vi "Collect_Info(V1.1).vi"(5 "HART ports":refnum<visa-resource-name>[](array[refnum]), 7 "485 Ports":refnum<visa-resource-name>[](array[refnum]), 10 "MODBUS Serial Parameters":T10={"Mode"=enum."RTU", "Default Slave Address"=111, "MODBUS timeout"=1000, "Baud Rate"=38400, "Parity"=0, "Flow Control"=0} {"Flow Control" items=["None", "XON/XOFF", "RTS/CTS", "XON/XOFF & RTS/CTS", "DTR/DSR", "XON/XOFF & DTR/DSR"]; "Parity" items=["None", "Odd", "Even", "Mark", "Space"]}) -> (1 "Read Completed":bool, 2 "Information":T11, 3 "Byte order":T7(ring))   [LabVIEW 2016]
uses:
  Controls/Control_Done.ctl
  Controls/Flow Tube Material.ctl
  Controls/mass flow unit codes.ctl
  Controls/Density Unit codes.ctl
  Controls/Temperature units.ctl
  Controls/Flow direction codes.ctl
  Controls/Information_tab_type.ctl
  Controls/Control_Sample.ctl
  OPC Server/MODBUS/MODBUS parameters type.ctl
  <vilib>/DeviceNet/VIAPI/subVIs/DnetIntfConfig.ctl
  OPC Server/Typedef/Array_of_Comm_mode_and_address_types.ctl
  OPC Server/Typedef/Comm_mode_and_address_type.ctl
  OPC Server/Typedef/Comm_mode_type_combo.ctl
  Controls/Control_EXIT.ctl
  Controls/ctrlCollectInfoStates.ctl
  Controls/ctrlCollectInfoData.ctl
  OPC Server/Protocol Class/Protocol.lvclass
  OPC Server/Typedef/comm_variable_definition.ctl
  OPC Server/MASTER_OPC.ctl
  OPC Server/Typedef/event var.ctl
  OPC Server/Typedef/Comm ui action type.ctl
  OPC Server/Typedef/Comm_State_enum.ctl
  OPC Server/Typedef/state var.ctl
  <vilib>/Utility/miscctls.llb/LVPointTypeDef.ctl
  OPC Server/MODBUS/MODBUS Class/MODBUS.lvclass
  C:/Application/Blackbox_US-Rabi--master/OPC Server/Protocol Class/Protocol.lvclass
  OPC Server/HART/HART Class/HART.lvclass
  OPC Server/Profibus/Profibus Class/Profibus.lvclass
  OPC Server/DeviceNET/DeviceNET Class/DeviceNET.lvclass
  OPC Server/Typedef/Protocol_enum_type.ctl
  <vilib>/DeviceNet/DeviceNetLIB.lvlib
panel:
  out "status":bool
  in  "Protocol selection\n(appended)":T1=[{"address"=111, "Mode"=0}, {"address"=0, "Mode"=2}] {"Mode" items=["MODBUS", "HART", ""]}
  in  "Done":T4
  in  "Read":T5
  in  "Batch Time":string
  in  "Pressure":string
  in  "Frequency":string
  in  "Test Gas":string
  in  "Stand Uncertainty":string
  in  "Customer PO":string
  in  "Fluid Temperature":string
  in  "Exit":T6
  in  "MDOT":string
  in  "Meter inlet static pressure (psia)":dbl
  in  "Fluid":string="H2O"
  in  "Product code*":string
  in  "Order number":string
  in  "Status *":enum32{"As found", "As left"}(radio)
  in  "Ref meter serial number*":string
  in  "Technician Name*":string
  in  "Customer Address":string
  in  "Customer Name":string
  in  "Interface Name":T8(ring)
  in  "DeviceNet Interface Configuration":T9={"interface MAC ID"=0, "baud rate"=enum."500000", "poll mode"=enum."Automatic"} {"interface MAC ID" max=63 step=1}
  in  "Profibus Baud rate":i32(listbox)=6
  in  "Profibus ResourceName":refnum<visa-resource-name>="PXI5::11::INSTR"
  in  "Test Comments":string
  out "Test date and time":string
  out "Meter Zero":string
  in  "Meter Nominal Flow Rate (kg/min)*":string
  in  "Meter Density Repeatability":string
  in  "Meter Density Accuracy":string
  in  "Meter Zero Stability (kg/min) *":string
  in  "Meter flow repeatability":string
  in  "Meter flow accuracy (%) *":string
  out "Frequency span":string
  out "Frequency flow rate":string
  out "Flow direction":T12 items=["Forward flow only", "Reverse flow only", "Bidirectiona flow", "Absolute forward/reverse", "Negate/Forward only", "Negate/Bidirectional"]
  out "Mass flow damping":string
  out "Mass flow cutoff":string
  out "Temperature Units":T13 items=["Degrees Celsius"=32, "Degrees Fahrenheit"=33, "Degrees Rankine"=34, "Degrees Kelvin"=35, ""=0]
  out "Density units":T14 items=["Specific gravity units"=90, "Grams/cubic centimeter"=91, "Kg/cubic meter"=92, "Pounds/US gallon"=93, "Pounds/cubic foot"=94, "Grams/milliliter"=95, "Kg/liter"=96, "Pounds/cubic inch"=98, "Short tons/cubic yard"=99, "Degrees Baume (heavy)"=102, "Degrees Baume (light)"=103, "Degrees API"=104]
  out "Mass flow units":T15 items=["Grams/second"=70, "Grams/minute"=71, "Grams/hour"=72, "Kg/second"=73, "Kg/minute"=74, "Kg/hour"=75, "Kg/day"=76, "Metric tons/minute"=77, "Metric tons/hour"=78, "Metric tons/day"=79, "Pounds/second"=80, "Pounds/minute"=81, "Pounds/hour"=82, "Pounds/day"=83, "Short tons/minute"=84, "Short tons/hour"=85, "Short tons/day"=86, "Long tons/hour"=87, "Long tons/day"=88, "Special"=253]
  out "Transmitter Model":string
  in  "Sensor Model #":string
  in  "Transmitter Serial Number":string
  out "Density Temp Coeff":string
  out "FD":string
  out "K2":string
  out "K1":string
  out "D2":string
  out "D1":string
  out "FCF":string
  in  "Temp Rating":string
  in  "Pressure Rating":string
  out "Sensor Serial Number":string
  out "Flow Tube Material":T16 items=["Hastelloy C-22"=3, "Monel"=4, "Tantalum"=5, "Titanium"=6, "316L Stainless Steel"=19, "Inconel"=23, "Unknown"=252, "Special"=253]
  in  "Size":string
  out "Header":string="CUSTOMER INFORMATION"
  # "Customer Information"
  # "*Required"
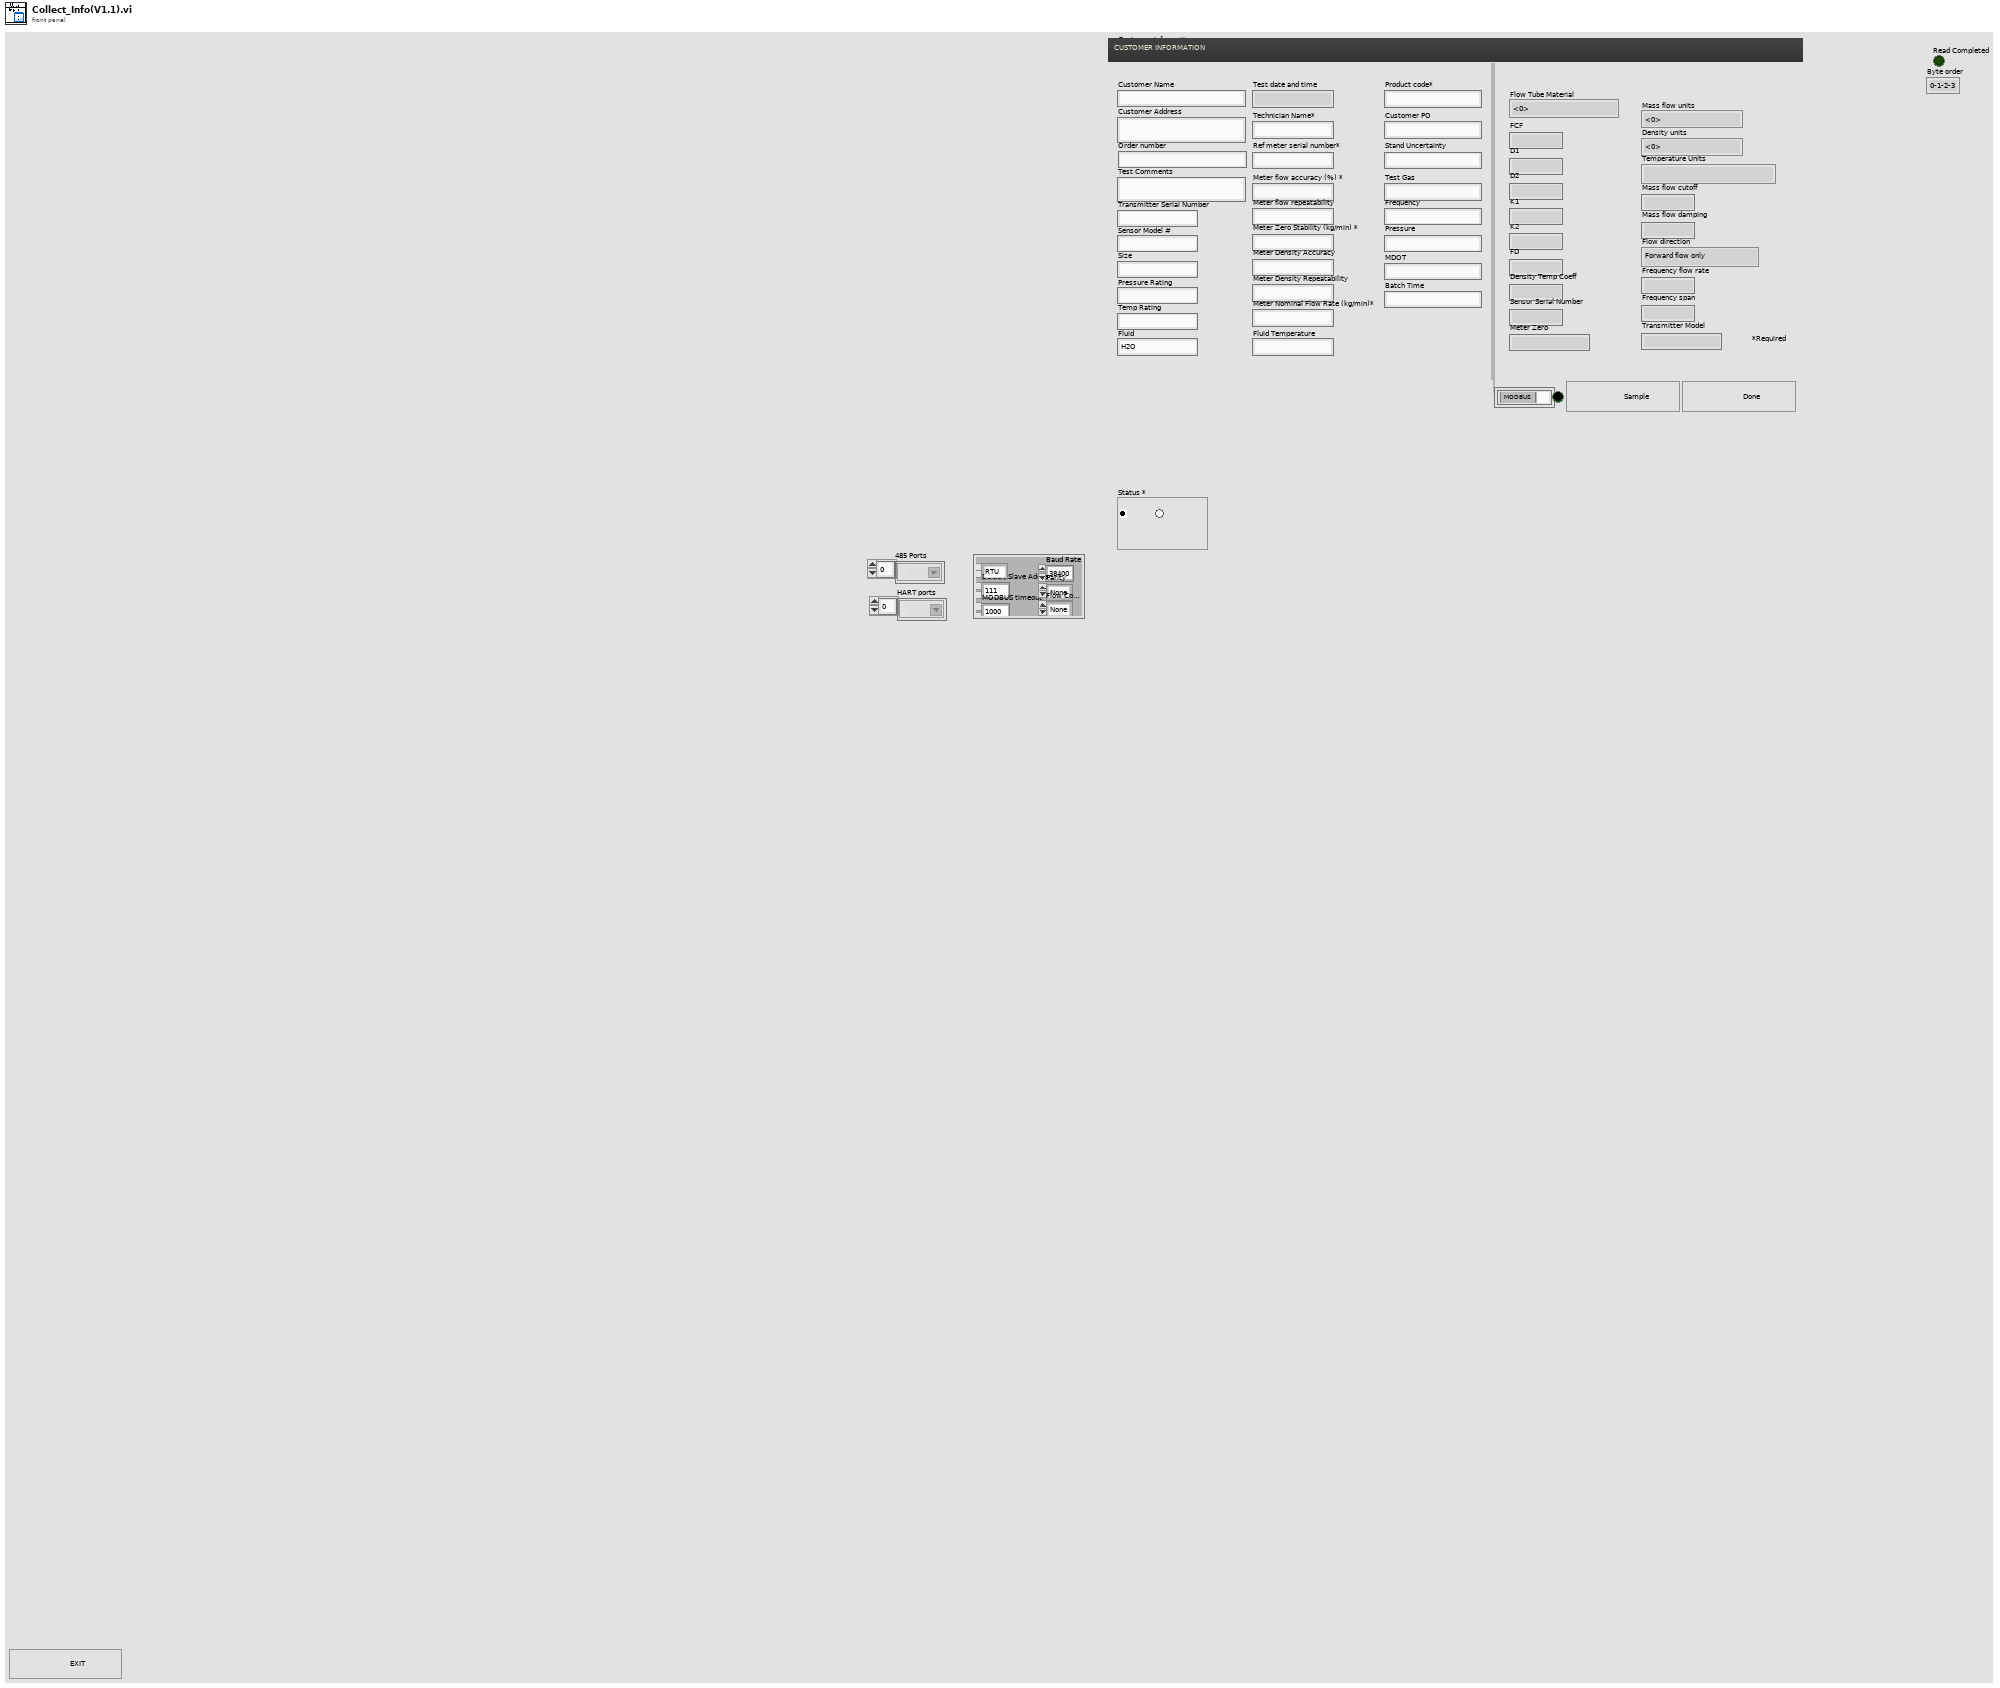
[diagram p1: front panel]
types:
  T1 = typedef "Array_of_Comm_mode_and_address_types.ctl" = T2[]
  T2 = typedef "Comm_mode_and_address_type.ctl" = cluster{"address":i32, "Mode":T3}
  T3 = typedef "Comm_mode_type_combo.ctl" = u16
  T4 = typedef "Control_Done.ctl" = bool
  T5 = typedef "Control_Sample.ctl" = bool
  T6 = typedef "Control_EXIT.ctl" = bool
  T7 = enum16{"0-1-2-3", "2-3-0-1", "1-0-3-2", "3-2-1-0"}
  T8 = enum16{"dnet0", "dnet1", "dnet2", "dnet3", "dnet4", "dnet5", "dnet6", "dnet7", "dnet8", "dnet9", "dnet10", "dnet11", "dnet12", "dnet13", "dnet14", "dnet15", "dnet16", "dnet17", "dnet18", "dnet19", "dnet20", "dnet21", "dnet22", "dnet23", "dnet24", "dnet25", "dnet26", "dnet27", "dnet28", "dnet29", "dnet30", "dnet31"}
  T9 = typedef "DeviceNetLIB.lvlib/DnetIntfConfig.ctl" = cluster{"interface MAC ID":u32, "baud rate":enum32{"125000", "250000", "500000"}, "poll mode":enum32{"Automatic", "Scanned", "Individual"}}
  T10 = typedef "MODBUS parameters type.ctl" = cluster{"Mode":enum16{"RTU", "ASCII"}, "Default Slave Address":u8, "MODBUS timeout":u32, "Baud Rate":u32, "Parity":u16, "Flow Control":u16}
  T11 = typedef "Information_tab_type.ctl" = cluster{"Test Date and Time, 1":string, "Test Comments,3":string, "Sensor Serial Number,6":string, "Sensor Model,7":string, "Size,8":string, "Material,9":string, "Press rating, 10":string, "Temp rating, 11":string, "FCF, 14":string, "D1, 15":string, "D2, 16":string, "K1, 17":string, "K2, 18":string, "FD, 19":string, "Density Temp Coeff, 20":string, "Transmitter Serial Number,23":string, "Transmitter Model Number,24":string, "Mass Flow Units, 25":string, "Density Units, 26":string, "Temperature Units, 27":string, "Mass Flow Cutoff, 28":string, "Mass Flow Damping, 29":string, "Flow Direction, 30":string, "Frequency Flow Rate, 31":string, "Frequency Span, 32":string, "Flow Accuracy, 35":string, "Flow Repeatability, 36":string, "Zero Stability, 37":string, "Density Accuracy, 38":string, "Density Repeatability, 39":string, "Nomincal Flow Rate, 41":string, "Meter Zero, 43":string, "Status, 45":string, "Customer name, 46":string, "Customer address, 47":string, "Sales order number, 48":string, "Technician Name, 49":string, "ref meter, 50":string, "product code,51":string, "fluid,52":string, "fluid temp,53":string, "Customer PO, 46":string, "Stand Uncertainty, 47":string, "Test Gas, 48":string, "Freq, 49":string, "Press, 50":string, "Mdot, 51":string, "Batch time, 52":string}
  T12 = typedef "Flow direction codes.ctl" = u16
  T13 = typedef "Temperature units.ctl" = u16
  T14 = typedef "Density Unit codes.ctl" = u16
  T15 = typedef "mass flow unit codes.ctl" = u16
  T16 = typedef "Flow Tube Material.ctl" = u16
  T17 = typedef "ctrlCollectInfoData.ctl" = cluster{"HART ports":refnum<visa-resource-name>[], "485 ports":refnum<visa-resource-name>[], "Byte order":enum16{"0-1-2-3", "2-3-0-1", "1-0-3-2", "3-2-1-0"}, "Read Complete?":bool, "ProtocolRef":refnum<vi>, "Data path":path, "ProtocolArray":refnum<class "Protocol.lvclass">[], "Protocol":refnum<class "Protocol.lvclass">, "Comm variable definitions":T18[], "Information":T11}
  T18 = typedef "comm_variable_definition.ctl" = cluster{"General Parameter name":string, "MODBUS Register":i32, "Profibus":cluster{"Friendly name":string, "PA":cluster{"Slot":i32, "Index":i32}, "DP":cluster{"Slot":i32, "Index":i32}, "Tag":string}, "Fieldbus":cluster{"Parameter name":string, "Fieldbus Block":string, "Fieldbus Tag":string}, "data type":enum16{"float", "UINT", "UINT32", "STRING"}, "DeviceNET":cluster{"ClassId":u16, "InstanceId":u16, "AttributeId":u8}, "Cluster":T2, "Length":i32}
  T19 = typedef "ctrlCollectInfoStates.ctl" = enum16{"WaitforEvents", "Init", "Read-Protocol", "Read-CommInfo", "Read-ByteOrder", "Read-FlowTubeMaterial", "Read-FlowCalibFactor", "Read-D1", "Read-D2", "Read-K1", "Read-K2", "Read-FD", "Read-DenTempCoeff", "Read-Srno", "Read-MassFlowUnits", "Read-DensityUnits", "Read-TempUnits", "Read-FlowCutoff", "Read-MassFlowDamping", "Read-FlowDirection", "Read-FreqFlowRate", "Read-FreqSpan", "Read-TransmitterModel", "Read-MeterZero", "ReadComplete", "Done&Close"}
  T20 = typedef "LVPointTypeDef.ctl" = cluster{"Horizontal":i16, "Vertical":i16}
  T21 = typedef "MASTER_OPC.ctl" = cluster{"Main event var":refnum<user-event>, "VIRef":refnum<vi>, "Data path":path, "Reads":i32, "total number of UUT":i32, "FF refnum":cluster{"Handle1":u32, "Handle2":u32}, "FF device id list":string[], "MODBUS resource name":refnum<visa-resource-name>, "MODBUS Serial Parameters":cluster{"Mode":enum16{"RTU", "ASCII"}, "Default Slave Address":u8, "MODBUS timeout":u32, "Baud Rate":u32, "Parity":u16, "Flow Control":u16}, "Profibus resource name":refnum<visa-resource-name>, "Profibus Communication ref.:":u8, "HART resource name":refnum<visa-resource-name>, "HART long addresses (array)":u8[][], "Comm relay session":refnum<k15>, "Comm UI event":refnum<user-event>, "Write Interval (s)":dbl, "DMM_QUEUE":refnum<queue>, "POWER_QUEUE":refnum<queue>, "\nTHERM_QUEUE":refnum<queue>, "\nCOMM_QUEUE":refnum<queue>, "TIMING_QUEUE":refnum<queue>, "MAIN_QUEUE":refnum<queue>, "Log path":path}
  T22 = typedef "Protocol_enum_type.ctl" = enum16{"None", "MODBUS", "HART", "Fieldbus", "Profibus DP", "Profibus PA", "DeviceNET", "USB"}
  T23 = cluster{"Current Path":path, "DataFiles Path":path, "ReportFiles Path":path, "SupportFiles Path":path, "ReportTemplate Path":path, "Sample_pulses_VIT_Path":path, "Sample_current_VIT_Path":path, "Sample_MODBUS_VIT_Path":path}
  T24 = typedef "CS_PB_DPV1_MSAC2_InitiateReqData.ctl" = cluster{"Communication ref.:":u8, "Send timeout:":u16, "Feat. supp. 1:":u8, "Feat. supp. 2:":u8, "Profile feat. supp. 1:":u8, "Profile feat. supp. 2:":u8, "Profile ID number:":u16, "Addional address parameter":cluster{"S-Type":bool, "S-Length:":u8, "D-Type":bool, "D-Length:":u8, "Data:":u8[]}}
  T25 = cluster{"U16":u16, "U32":u32, "float":sgl, "string":string}
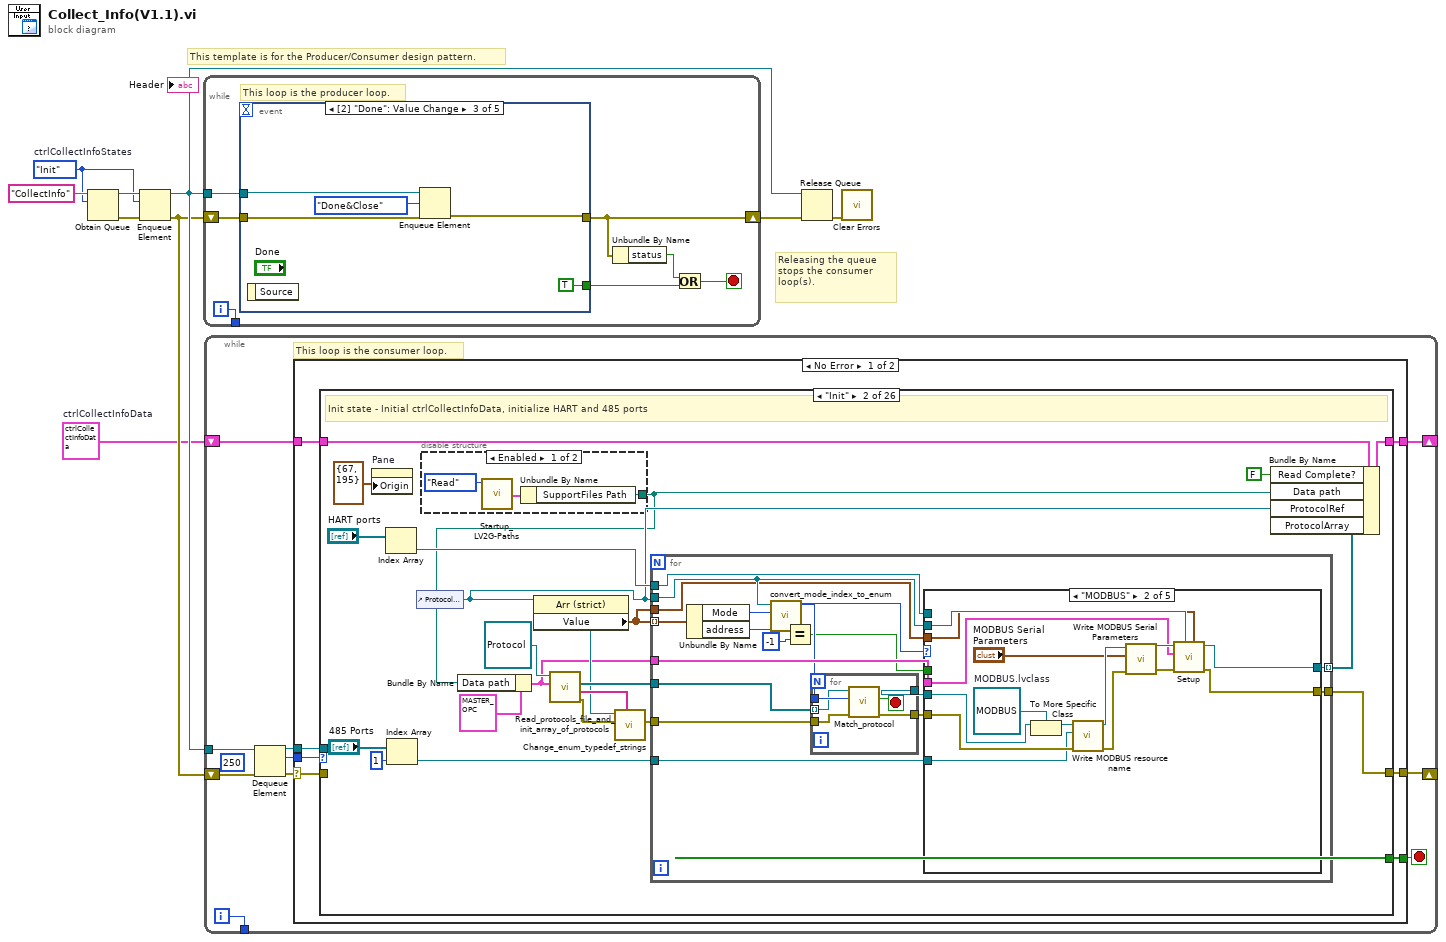
[diagram p0: block diagram]
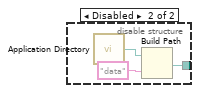
[diagram p3: hidden frame]
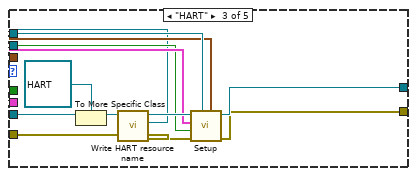
[diagram p5: hidden frame]
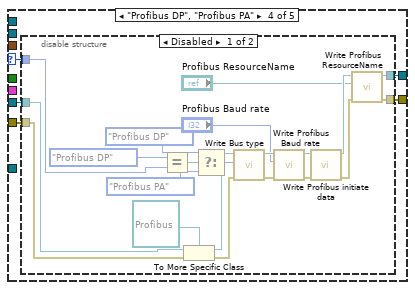
[diagram p6: hidden frame]
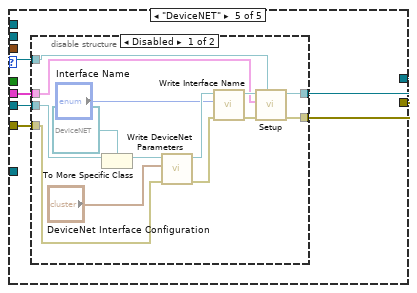
[diagram p8: hidden frame]
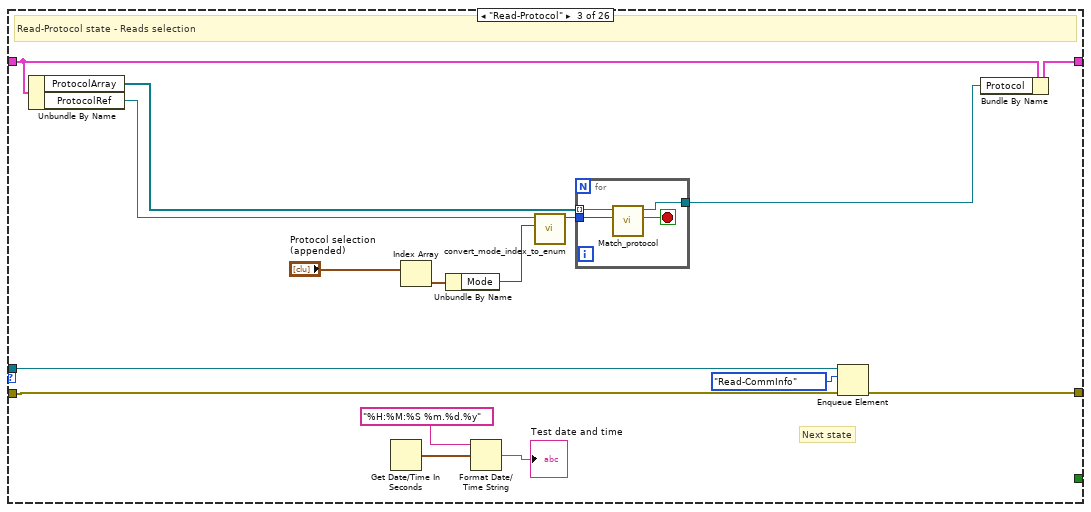
[diagram p10: hidden frame]
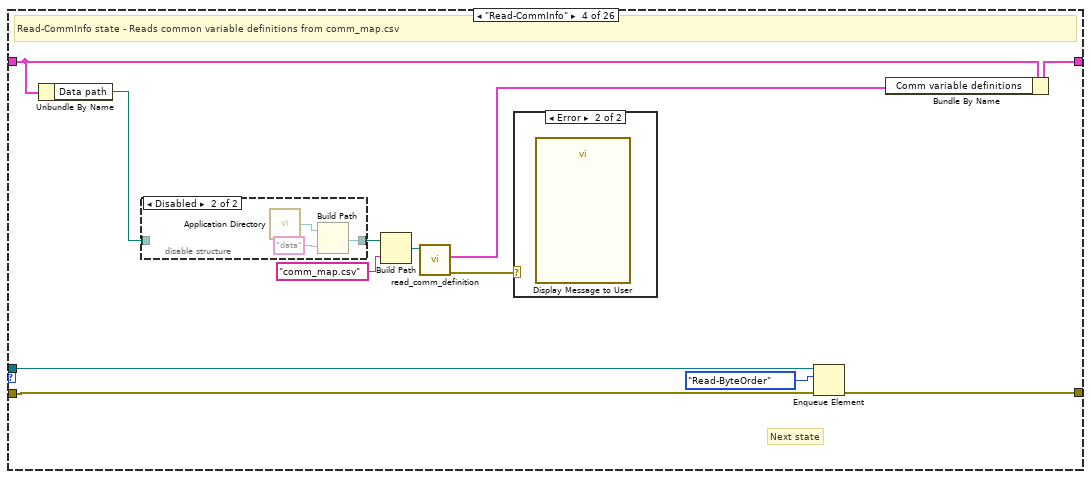
[diagram p11: hidden frame]
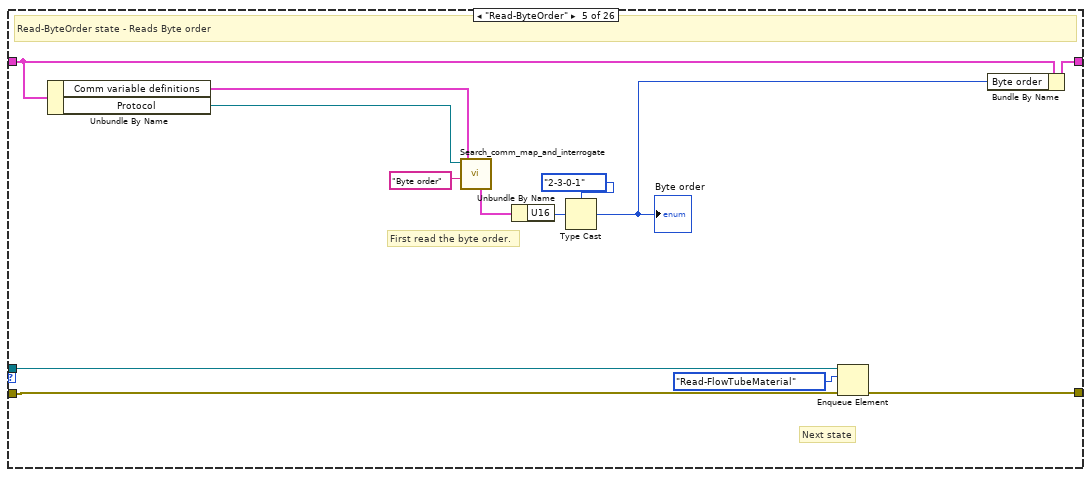
[diagram p14: hidden frame]
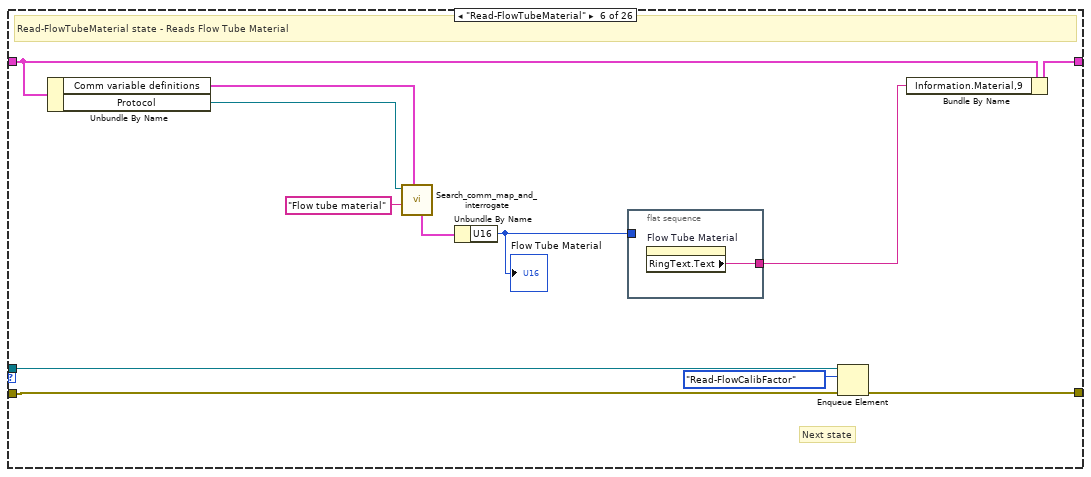
[diagram p15: hidden frame]
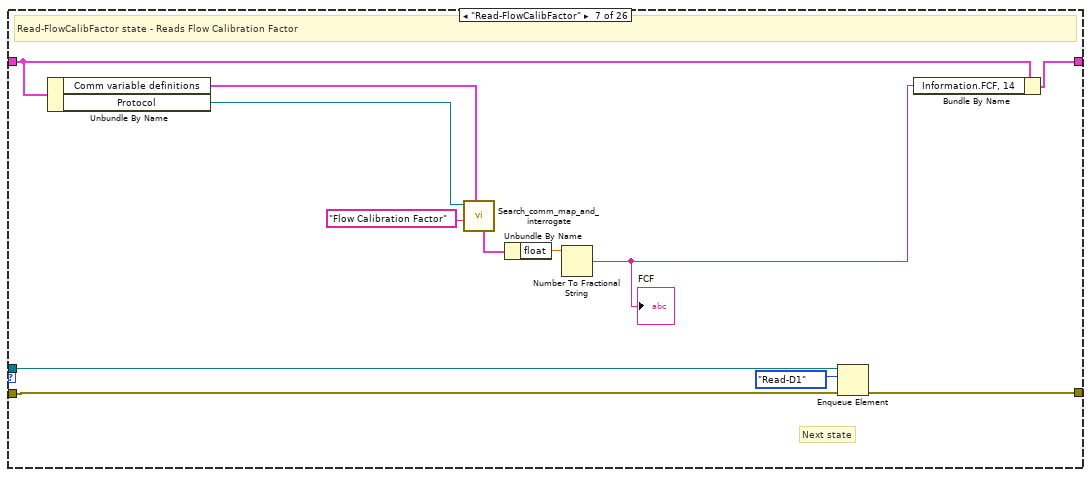
[diagram p16: hidden frame]
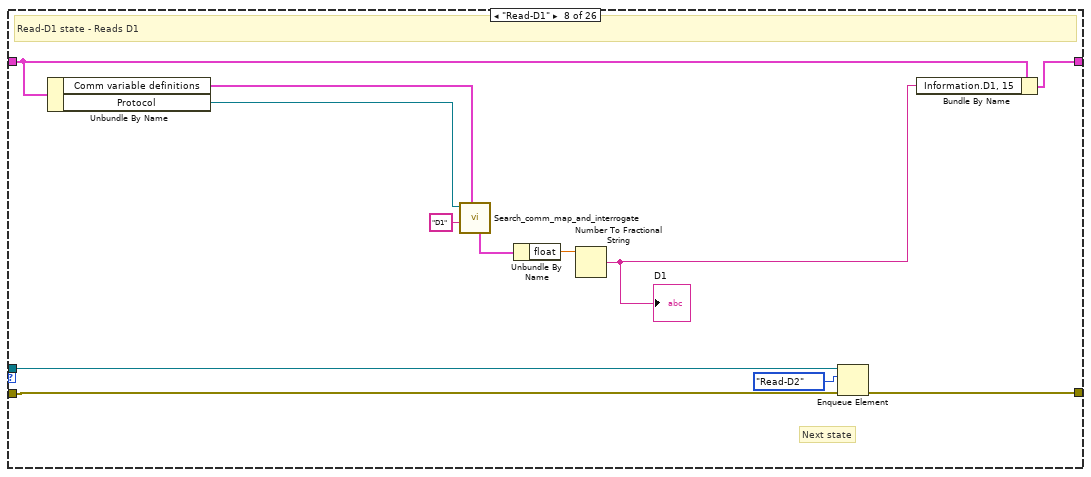
[diagram p17: hidden frame]
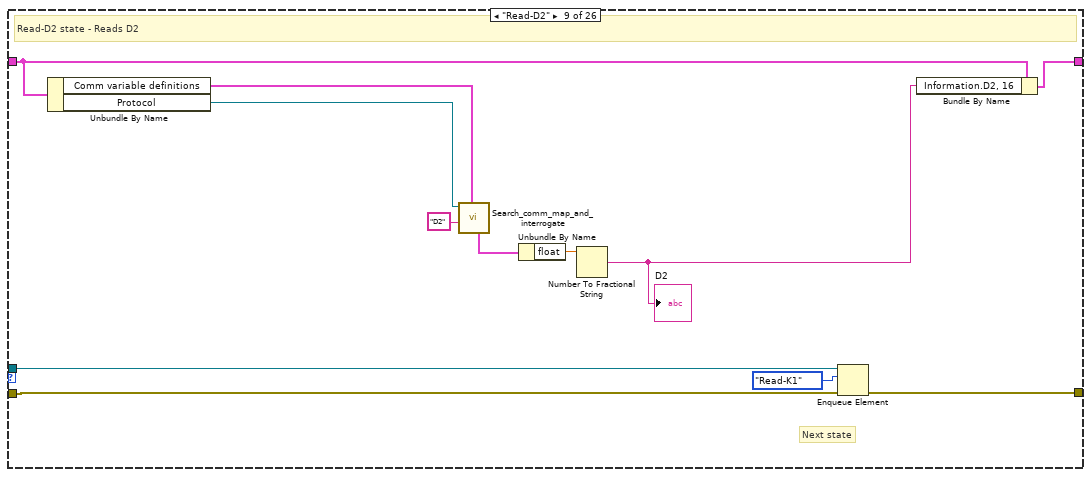
[diagram p18: hidden frame]
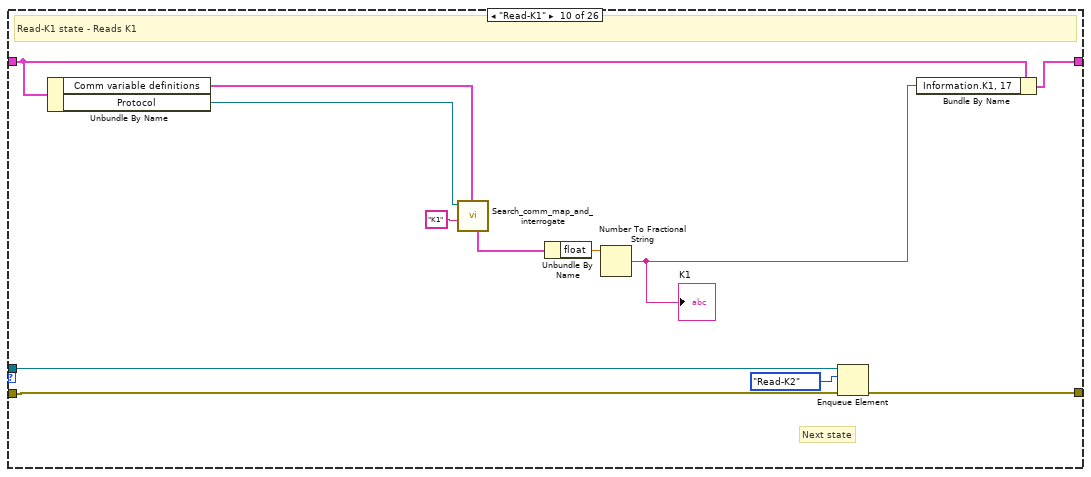
[diagram p19: hidden frame]
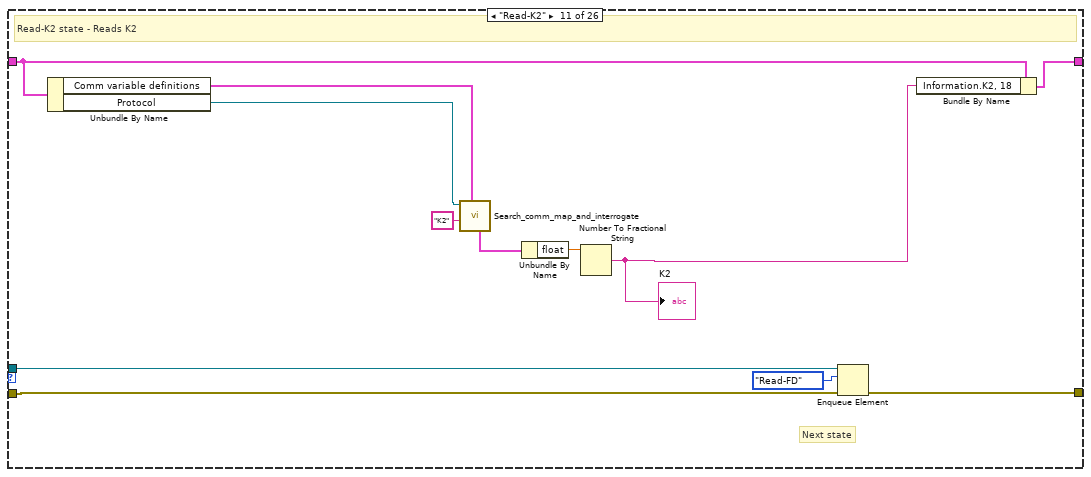
[diagram p20: hidden frame]
diagram:
  w1 = T17 {"HART ports"=[], "485 ports"=[], "Byte order"=enum."0-1-2-3", "Read Complete?"=FALSE, "ProtocolRef"=refnum, "Data path"=path "", "ProtocolArray"=[], "Protocol"=refnum, "Comm variable definitions"=[], "Information"={"Test Date and Time, 1"="", "Test Comments,3"="", "Sensor Serial Number,6"="", "Sensor Model,7"="", "Size,8"="", "Material,9"="", "Press rating, 10"="", "Temp rating, 11"="", "FCF, 14"="", "D1, 15"="", "D2, 16"="", "K1, 17"="", "K2, 18"="", "FD, 19"="", "Density Temp Coeff, 20"="", "Transmitter Serial Number,23"="", "Transmitter Model Number,24"="", "Mass Flow Units, 25"="", "Density Units, 26"="", "Temperature Units, 27"="", "Mass Flow Cutoff, 28"="", "Mass Flow Damping, 29"="", "Flow Direction, 30"="", "Frequency Flow Rate, 31"="", "Frequency Span, 32"="", "Flow Accuracy, 35"="", "Flow Repeatability, 36"="", "Zero Stability, 37"="", "Density Accuracy, 38"="", "Density Repeatability, 39"="", "Nomincal Flow Rate, 41"="", "Meter Zero, 43"="", "Status, 45"="", "Customer name, 46"="", "Customer address, 47"="", "Sales order number, 48"="", "Technician Name, 49"="", "ref meter, 50"="", "product code,51"="", "fluid,52"="", "fluid temp,53"="", "Customer PO, 46"="", "Stand Uncertainty, 47"="", "Test Gas, 48"="", "Freq, 49"="", "Press, 50"="", "Mdot, 51"="", "Batch time, 52"=""}}  # ctrlCollectInfoData
  w2 = ctrlCollectInfoStates."Init"  # ctrlCollectInfoStates
  # "This template is for the Producer/Consumer design pattern."
  # "Releasing the queue stops the consumer loop(s)."
  n1 = Obtain Queue(name (unnamed)="CollectInfo", element data type=w2) -> (queue out=w9:refnum<queue>, error out=w6:errorcluster)  [unwired: 3 in, 1 out]
  n2 = Enqueue Element(queue=w9, element=w2, error in (no error)=w6) -> (queue out=w4:refnum<queue>, error out=w3:errorcluster)  [unwired: 1 in, 1 out]
  n3 = while {
    tunnel: w4 -> [w16]
    tunnel: [w15] -> _
    shift-right: [w11] -> w5
    shift-left: w3 -> [w14]
    i -> [w15]
    stop <- w12 stop-if-true
    # "This loop is the producer loop."
    n4 = event shown="[2] \"Done\": Value Change" {
      selector: _ -> [_ _ _ _ _]
      dyn-events: _ -> [_ _ _ _ _]
      timeout: _ -> [_ _ _ _ _]
      tunnel: w16 -> [w17 w22 w26 _ _]
      tunnel: w14 -> [w20 w24 w29 w34 w39]
      tunnel: [w19 w23 w28 w34 w39] -> w11
      tunnel: [_ _ TRUE ("T button?") w31 w35] -> w10
      event Value Change {
        n5 = event-data() -> ()  [unwired: 1 in, 1 out]
        n6 = Enqueue Element(queue=w17, element=ctrlCollectInfoStates."Init" ("ctrlCollectInfoStates"), error in (no error)=w20) -> (error out=w19:errorcluster)  [unwired: 1 in, 2 out]
      }
      event Value Change {
        n7 = event-data() -> ()  [unwired: 1 in, 1 out]
        n8 = Enqueue Element(queue=w22, element=ctrlCollectInfoStates."Read-Protocol" ("ctrlCollectInfoStates"), error in (no error)=w24) -> (error out=w23:errorcluster)  [unwired: 1 in, 2 out]
      }
      event Value Change {
        n9 = event-data() -> ()  [unwired: 1 in, 1 out]
        n10 = Enqueue Element(queue=w26, element=ctrlCollectInfoStates."Done&Close" ("ctrlCollectInfoStates"), error in (no error)=w29) -> (error out=w28:errorcluster)  [unwired: 1 in, 2 out]
      }
      event Panel Close? {
        (unwired) "Cancel" ("F button name (\"Cancel\")")
        n11 = event-data() -> ()  [unwired: 1 in, 1 out]
        n12 = Two Button Dialog(message="Quitting will Abort all running program\nAre you sure you want to exit?", 2:"Quit" ("T button name (\"OK\")")) -> (T button?=w31:bool)  [unwired: 1 in]
        n13 = Not(x=w31) -> (.not. x?=w30:bool)
        n14 = event-data("Discard?"=w30) -> ()  [unwired: 1 in, 1 out]
      }
      event Value Change {
        n15 = event-data() -> ()  [unwired: 1 in, 1 out]
        n16 = Two Button Dialog(message="Quitting will Abort all running program\nAre you sure you want to exit?", 1:"Cancel" ("F button name (\"Cancel\")"), 2:"Quit" ("T button name (\"OK\")")) -> (T button?=w35:bool)
      }
    }
    n17 = Unbundle By Name(w11) -> ("status"=w13:bool)
    n18 = Or(x=w13, y=w10) -> (x .or. y?=w12:bool)
  }
  n19 = while {
    tunnel: w4 -> [w49]
    shift-right: [w44] -> _
    shift-left: w1 -> [w45]
    shift-right: [w41] -> _
    shift-left: w3 -> [w42]
    tunnel: [w40] -> _
    i -> [w40]
    stop <- w46 stop-if-true
    (unwired) 250 ("timeout in ms (-1)")
    # "This loop is the consumer loop."
    n20 = Dequeue Element(queue=w49, error in (no error)=w42) -> (queue out=w43:refnum<queue>, element=w47:T19, error out=w48:errorcluster)  [unwired: 1 in, 1 out]
    n21 = case shown="No Error" w48 {
      selector: w48 -> [w51 w518]
      tunnel: w47 -> [w54 _]
      tunnel: [w50 FALSE] -> w46
      tunnel: w45 -> [w55 w519]
      tunnel: [w56 w519] -> w44
      tunnel: w43 -> [w53 _]
      tunnel: [w52 w517] -> w41
      frame No Error {
        n22 = case shown="\"Init\"" w54 {
          tunnel: [w57 w71 w201 w214 w224 w246 w259 w271 w283 w295 w307 w319 w331 w343 w355 w368 w381 w394 w406 w418 w431 w443 w455 w469 w476 w488] -> w56
          tunnel: w55 -> [w57 w72 w193 w207 w225 w242 w255 w267 w279 w291 w303 w315 w327 w339 w351 w364 w377 w390 w402 w414 w427 w439 w451 w464 w471 w489]
          tunnel: w53 -> [_ _ w200 w212 w234 w245 w258 w270 w282 w294 w306 w318 w330 w342 w354 w367 w380 w393 w405 w417 w430 w442 w454 w468 w475 _]
          tunnel: [w58 w63 w198 w210 w232 w243 w256 w268 w280 w292 w304 w316 w328 w340 w352 w365 w378 w391 w403 w415 w428 w440 w452 w466 w473 w486] -> w52
          tunnel: w51 -> [w58 _ w199 w211 w233 w244 w257 w269 w281 w293 w305 w317 w329 w341 w353 w366 w379 w392 w404 w416 w429 w441 w453 w467 w474 w486]
          tunnel: [_ _ _ _ _ _ _ _ _ _ _ _ _ _ _ _ _ _ _ _ _ _ _ _ _ TRUE] -> w50
          frame "WaitforEvents", Default {
            # "WaitforEvents state - do nothing, just wait for command from producer loop"
          }
          frame "Init" {
            # "Init state - Initial ctrlCollectInfoData, initialize HART and 485 ports"
            n23 = property on="Pane" class="Pane"("Origin"=T20 {"Horizontal"=67, "Vertical"=195}) -> ()  [unwired: 2 in, 2 out]
            n24 = Index Array(array="HART ports") -> (element=w66:refnum<visa-resource-name>)  [unwired: 1 in]
            n25 = Index Array(array="485 Ports", index=1) -> (element=w65:refnum<visa-resource-name>)
            n26 = control-ref of="Protocol selection\n(appended)"() -> (w64:refnum<vi>)
            n27 = disable-structure shown="Enabled" {
              disable-tunnel: [w80 w83] -> w59
              frame Enabled {
                n28 = call "Startup_LV2G-Paths.vi"("Action"=enum16{"Read", "Write"}."Read") -> ("Paths"=w82:T23)  [unwired: 9 in, 1 out]
                n29 = Unbundle By Name(w82) -> ("SupportFiles Path"=w80:path)
              }
              frame Disabled {
                n30 = call <vilib>:"Application Directory.vi"() -> ("Application Directory"=w84:path)
                n31 = Build Path(base path=w84, name or relative path="data") -> (appended path=w83:path)
              }
            }
            n32 = Bundle By Name(cluster=T21 {"Main event var"=refnum, "VIRef"=refnum, "Data path"=path "", "Reads"=0, "total number of UUT"=0, "FF refnum"={"Handle1"=0, "Handle2"=0}, "FF device id list"=[], "MODBUS resource name"="", "MODBUS Serial Parameters"={"Mode"=enum."RTU", "Default Slave Address"=0, "MODBUS timeout"=0, "Baud Rate"=0, "Parity"=0, "Flow Control"=0}, "Profibus resource name"="", "Profibus Communication ref.:"=0, "HART resource name"="", "HART long addresses (array)"=[], "Comm relay session"="", "Comm UI event"=refnum, "Write Interval (s)"=5.0, "DMM_QUEUE"=refnum, "POWER_QUEUE"=refnum, "\nTHERM_QUEUE"=refnum, "\nCOMM_QUEUE"=refnum, "TIMING_QUEUE"=refnum, "MAIN_QUEUE"=refnum, "Log path"=path ""} ("Comm master cluster"), "Data path"=w59) -> (w60:T21)
            n33 = property class="Arr (strict)"(reference=w64) -> ("Value"=w73:T1)  [unwired: 1 in, 2 out]
            n34 = call-dynamic "Read_protocols_file_and_init_array_of_protocols.vi"("Comm master cluster"=w60, "Protocol in"=refnum<class "Protocol.lvclass"> refnum) -> ("error out"=w77:errorcluster, "Array of configured protocols"=w76:string[], "Array of Protocols out"=w75:refnum<class "Protocol.lvclass">[])  [unwired: 6 in, 1 out]
            n35 = call "Change_enum_typedef_strings.vi"("Strings []"=w76, "error in (no error)"=w77, "protocol selection ref"=w64) -> ("error out"=w78:errorcluster)  [unwired: 8 in]
            n36 = for {
              tunnel: w75 -> [w96]
              tunnel: [w102] -> w70 mode=indexing
              tunnel: [w101] -> w63
              tunnel: w64 -> [w99]
              tunnel: w78 -> [w93]
              tunnel: w60 -> [w100]
              tunnel: w73 -> [w98] mode=indexing
              tunnel: w73 -> [w88]
              tunnel: w66 -> [w87]
              tunnel: w65 -> [w86]
              n37 = Unbundle By Name(w98) -> ("Mode"=w97:T3, "address"=w91:i32)
              n38 = call "convert_mode_index_to_enum.vi"("index"=w97, "CtlRef"=w99) -> ("Protocol enum"=w92:T22)  [unwired: 6 in, 3 out]
              n39 = Equal?(x=w91, y=-1) -> (x = y?=w89:bool)
              n40 = for {
                tunnel: [w108] -> w95
                tunnel: [w106] -> w94
                tunnel: w92 -> [w105]
                tunnel: w96 -> [w104] mode=indexing
                tunnel: w93 -> [w103]
                stop <- w107 stop-if-true
                n41 = call-dynamic "Match_protocol.vi"("error in (no error)"=w103, "Protocol type"=w105, "Protocol in"=w104) -> ("error out"=w106:errorcluster, "Match"=w107:bool, "Protocol out"=w108:refnum<class "Protocol.lvclass">)  [unwired: 6 in]
              }
              n42 = case shown="\"MODBUS\"" w92 {
                selector: w92 -> [_ _ _ w140 _]
                tunnel: w95 -> [w110 w125 w138 w143 w171]
                tunnel: [w110 w123 w134 w139 w170] -> w102
                tunnel: [w109 w116 w131 w142 w169] -> w101
                tunnel: w94 -> [w109 w115 w136 w141 w168]
                tunnel: w100 -> [_ w114 w133 _ w167]
                tunnel: w99 -> [_ w113 w130 _ w166]
                tunnel: w89 -> [_ _ w128 _ _]
                tunnel: w88 -> [_ w112 w127 _ _]
                tunnel: w87 -> [_ _ w126 _ _]
                tunnel: w86 -> [_ w111 _ _ _]
                frame "None", Default {
                }
                frame "MODBUS" {
                  w124 = refnum<class "MODBUS.lvclass"> refnum  # MODBUS.lvclass
                  n43 = To More Specific Class(target class=w124, reference=w125) -> (specific class reference=w122:refnum<class "MODBUS.lvclass">)  [unwired: 1 in, 1 out]
                  n44 = call-dynamic "Write MODBUS resource name.vi"("error in (no error)"=w115, "MODBUS resource name"=w111, "MODBUS in"=w122) -> ("error out"=w121:errorcluster, "MODBUS out"=w120:refnum<class "MODBUS.lvclass">)  [unwired: 7 in]
                  n45 = call-dynamic "Write MODBUS Serial Parameters.vi"("error in (no error)"=w121, "MODBUS Serial Parameters"="MODBUS Serial Parameters", "MODBUS in"=w120) -> ("error out"=w117:errorcluster, "MODBUS out"=w118:refnum<class "MODBUS.lvclass">)  [unwired: 7 in]
                  n46 = call-dynamic "Setup.vi"("Protocol selection\n(appended)"=w112, "protocol selection ref"=w113, "error in (no error)"=w117, "Comm master cluster in"=w114, "MODBUS in"=w118) -> ("error out"=w116:errorcluster, "MODBUS out"=w123:refnum<class "MODBUS.lvclass">)  [unwired: 5 in]
                }
                frame "HART" {
                  n47 = To More Specific Class(target class=refnum<class "HART.lvclass"> refnum ("HART.lvclass"), reference=w138) -> (specific class reference=w137:refnum<class "HART.lvclass">)  [unwired: 1 in, 1 out]
                  n48 = call-dynamic "Write HART resource name.vi"("error in (no error)"=w136, "HART resource name"=w126, "HART in"=w137) -> ("error out"=w132:errorcluster, "HART out"=w135:refnum<class "HART.lvclass">)  [unwired: 7 in]
                  n49 = call-dynamic "Setup.vi"("Protocol selection\n(appended)"=w127, "protocol selection ref"=w130, "error in (no error)"=w132, "search"=w128, "Comm master cluster in"=w133, "HART in"=w135) -> ("error out"=w131:errorcluster, "HART out"=w134:refnum<class "HART.lvclass">)  [unwired: 4 in]
                }
                frame "Profibus DP", "Profibus PA" {
                  n50 = disable-structure shown="Disabled" {
                    disable-tunnel: w143 -> [w164 _]
                    disable-tunnel: [w160 _] -> w142
                    disable-tunnel: w141 -> [w154 _]
                    disable-tunnel: w140 -> [w152 _]
                    disable-tunnel: [w144 _] -> w139
                    frame Disabled {
                      n51 = Equal?(x=Protocol_enum_type."Profibus DP" ("Protocols"), y=w152) -> (x = y?=w151:bool)
                      n52 = To More Specific Class(target class=refnum<class "Profibus.lvclass"> refnum ("Profibus.lvclass"), reference=w164, error in=w154) -> (specific class reference=w156:refnum<class "Profibus.lvclass">, error out=w155:errorcluster)
                      n53 = Select(t=enum16{"Profibus DP", "Profibus PA"}."Profibus DP" ("Bus type"), s=w151, f=enum16{"Profibus DP", "Profibus PA"}."Profibus PA" ("Bus type")) -> (s? t:f=w148:enum16{"Profibus DP", "Profibus PA"})
                      n54 = call-dynamic "Write Bus type.vi"("error in (no error)"=w155, "Bus type"=w148, "Profibus in"=w156) -> ("error out"=w163:errorcluster, "Profibus out"=w159:refnum<class "Profibus.lvclass">)  [unwired: 7 in]
                      n55 = call-dynamic "Write Profibus Baud rate.vi"("error in (no error)"=w163, "Profibus Baud rate"="Profibus Baud rate", "Profibus in"=w159) -> ("error out"=w162:errorcluster, "Profibus out"=w158:refnum<class "Profibus.lvclass">)  [unwired: 7 in]
                      n56 = call-dynamic "Write Profibus initiate data.vi"("error in (no error)"=w162, "Profibus in"=w158) -> ("error out"=w161:errorcluster, "Profibus out"=w157:refnum<class "Profibus.lvclass">, "Initiate data"=w146:T24)  [unwired: 7 in]
                      n57 = call-dynamic "Write Profibus ResourceName.vi"("error in (no error)"=w161, "Profibus ResourceName"="Profibus ResourceName", "Profibus in"=w157) -> ("error out"=w160:errorcluster, "Profibus out"=w144:refnum<class "Profibus.lvclass">)  [unwired: 7 in]
                    }
                    frame Enabled {
                    }
                  }
                }
                frame "DeviceNET" {
                  n58 = disable-structure shown="Disabled" {
                    disable-tunnel: w171 -> [w185 _]
                    disable-tunnel: [w184 _] -> w170
                    disable-tunnel: [w183 _] -> w169
                    disable-tunnel: w168 -> [w177 _]
                    disable-tunnel: w167 -> [w173 _]
                    disable-tunnel: w166 -> [w172 _]
                    frame Disabled {
                      n59 = To More Specific Class(target class=refnum<class "DeviceNET.lvclass"> refnum ("DeviceNET.lvclass"), reference=w185) -> (specific class reference=w174:refnum<class "DeviceNET.lvclass">)  [unwired: 1 in, 1 out]
                      n60 = call-dynamic "Write DeviceNet Parameters.vi"("error in (no error)"=w177, "DeviceNet Interface Configuration"="DeviceNet Interface Configuration", "DeviceNET in"=w174) -> ("error out"=w176:errorcluster, "DeviceNET out"=w181:refnum<class "DeviceNET.lvclass">)  [unwired: 7 in]
                      n61 = call-dynamic "Write Interface Name.vi"("error in (no error)"=w176, "Interface Name"="Interface Name", "DeviceNET in"=w181) -> ("error out"=w175:errorcluster, "DeviceNET out"=w180:refnum<class "DeviceNET.lvclass">)  [unwired: 7 in]
                      n62 = call-dynamic "Setup.vi"("protocol selection ref"=w172, "error in (no error)"=w175, "Comm master cluster in"=w173, "DeviceNET in"=w180) -> ("error out"=w183:errorcluster, "DeviceNET out"=w184:refnum<class "DeviceNET.lvclass">)  [unwired: 6 in]
                    }
                    frame Enabled {
                    }
                  }
                }
              }
            }
            n63 = Bundle By Name(cluster=w72, "Read Complete?"=FALSE, "Data path"=w59, "ProtocolRef"=w64, "ProtocolArray"=w70) -> (w71:T17)
          }
          frame "Read-Protocol" {
            # "Next state"
            # "Read-Protocol state - Reads selection"
            n64 = Unbundle By Name(w193) -> ("ProtocolArray"=w192:refnum<class "Protocol.lvclass">[], "ProtocolRef"=w191:refnum<vi>)
            n65 = Get Date/Time In Seconds() -> (seconds since 1Jan1904=w189:timestamp)
            n66 = Index Array(array="Protocol selection\n(appended)") -> (element=w196:T2)  [unwired: 1 in]
            n67 = Unbundle By Name(w196) -> ("Mode"=w195:T3)
            n68 = Format Date/Time String(time format string (%c)="%H:%M:%S %m.%d.%y", seconds (now)=w189) -> (date/time string=→"Test date and time":string)  [unwired: 1 in]
            n69 = call "convert_mode_index_to_enum.vi"("index"=w195, "CtlRef"=w191) -> ("Protocol enum"=w194:T22)  [unwired: 6 in, 3 out]
            n70 = for {
              tunnel: w194 -> [w205]
              tunnel: w192 -> [w204] mode=indexing
              tunnel: [w202] -> w190
              stop <- w203 stop-if-true
              n71 = call-dynamic "Match_protocol.vi"("Protocol type"=w205, "Protocol in"=w204) -> ("Match"=w203:bool, "Protocol out"=w202:refnum<class "Protocol.lvclass">)  [unwired: 7 in, 1 out]
            }
            n72 = Enqueue Element(queue=w200, element=ctrlCollectInfoStates."Read-CommInfo" ("ctrlCollectInfoStates"), error in (no error)=w199) -> (error out=w198:errorcluster)  [unwired: 1 in, 2 out]
            n73 = Bundle By Name(cluster=w193, "Protocol"=w190) -> (w201:T17)
          }
          frame "Read-CommInfo" {
            # "Next state"
            # "Read-CommInfo state - Reads common variable definitions from comm_map.csv"
            n74 = Unbundle By Name(w207) -> ("Data path"=w206:path)
            n75 = disable-structure shown="Disabled" {
              disable-tunnel: [w218 w219] -> w208
              disable-tunnel: w206 -> [w218 _]
              frame Enabled {
              }
              frame Disabled {
                n76 = call <vilib>:"Application Directory.vi"() -> ("Application Directory"=w220:path)
                n77 = Build Path(base path=w220, name or relative path="data") -> (appended path=w219:path)
              }
            }
            n78 = Build Path(base path=w208, name or relative path="comm_map.csv") -> (appended path=w217:path)
            n79 = call "read_comm_definition.vi"("file path (dialog if empty)"=w217) -> ("error out"=w215:errorcluster, "Comm variable definitions"=w213:T18[])  [unwired: 8 in, 1 out]
            n80 = case shown="Error" w215 {
              frame No Error {
              }
              frame Error {
                n81 = call "Display Message to User"() -> ()  [unwired: 10 in, 2 out]
              }
            }
            n82 = Enqueue Element(queue=w212, element=ctrlCollectInfoStates."Read-ByteOrder" ("ctrlCollectInfoStates"), error in (no error)=w211) -> (error out=w210:errorcluster)  [unwired: 1 in, 2 out]
            n83 = Bundle By Name(cluster=w207, "Comm variable definitions"=w213) -> (w214:T17)
          }
          frame "Read-ByteOrder" {
            # "First read the byte order."
            # "Next state"
            # "Read-ByteOrder state - Reads Byte order"
            n84 = Unbundle By Name(w225) -> ("Comm variable definitions"=w226:T18[], "Protocol"=w227:refnum<class "Protocol.lvclass">)
            n85 = call "Search_comm_map_and_interrogate.vi"("array of registers"=w226, "Register name"="Byte order", "Protocol in"=w227) -> ("output cluster"=w229:T25)  [unwired: 6 in, 2 out]
            n86 = Unbundle By Name(w229) -> ("U16"=w228:u16)
            n87 = Type Cast(type=T7."2-3-0-1" ("Byte order"), x=w228) -> (*(type *) &x=w223:T7)
            "Byte order" <- w223
            n88 = Enqueue Element(queue=w234, element=ctrlCollectInfoStates."Read-FlowTubeMaterial" ("ctrlCollectInfoStates"), error in (no error)=w233) -> (error out=w232:errorcluster)  [unwired: 1 in, 2 out]
            n89 = Bundle By Name(cluster=w225, "Byte order"=w223) -> (w224:T17)
          }
          frame "Read-FlowTubeMaterial" {
            # "Next state"
            # "Read-FlowTubeMaterial state - Reads Flow Tube Material"
            n90 = Unbundle By Name(w242) -> ("Comm variable definitions"=w236:T18[], "Protocol"=w238:refnum<class "Protocol.lvclass">)
            n91 = call "Search_comm_map_and_interrogate.vi"("array of registers"=w236, "Register name"="Flow tube material", "Protocol in"=w238) -> ("output cluster"=w239:T25)  [unwired: 6 in, 2 out]
            n92 = Unbundle By Name(w239) -> ("U16"=w241:u16)
            "Flow Tube Material" <- w241
            n93 = flat-sequence {
              tunnel: [w247] -> w237
              tunnel: w241 -> [_]
              frame #0 {
                n94 = property on="Flow Tube Material" class="Ring (strict)"() -> ("RingText.Text"=w247:string)  [unwired: 2 in, 2 out]
              }
            }
            n95 = Enqueue Element(queue=w245, element=ctrlCollectInfoStates."Read-FlowCalibFactor" ("ctrlCollectInfoStates"), error in (no error)=w244) -> (error out=w243:errorcluster)  [unwired: 1 in, 2 out]
            n96 = Bundle By Name(cluster=w242, "Information.Material,9"=w237) -> (w246:T17)
          }
          frame "Read-FlowCalibFactor" {
            # "Next state"
            # "Read-FlowCalibFactor state - Reads Flow Calibration Factor"
            n97 = Unbundle By Name(w255) -> ("Comm variable definitions"=w250:T18[], "Protocol"=w249:refnum<class "Protocol.lvclass">)
            n98 = call "Search_comm_map_and_interrogate.vi"("array of registers"=w250, "Register name"="Flow Calibration Factor", "Protocol in"=w249) -> ("output cluster"=w253:T25)  [unwired: 6 in, 2 out]
            n99 = Unbundle By Name(w253) -> ("float"=w252:sgl)
            n100 = Number To Fractional String(number=w252) -> (F-format string=w251:string)  [unwired: 3 in]
            "FCF" <- w251
            n101 = Enqueue Element(queue=w258, element=ctrlCollectInfoStates."Read-D1" ("ctrlCollectInfoStates"), error in (no error)=w257) -> (error out=w256:errorcluster)  [unwired: 1 in, 2 out]
            n102 = Bundle By Name(cluster=w255, "Information.FCF, 14"=w251) -> (w259:T17)
          }
          frame "Read-D1" {
            # "Next state"
            # "Read-D1 state - Reads D1"
            n103 = Unbundle By Name(w267) -> ("Comm variable definitions"=w263:T18[], "Protocol"=w262:refnum<class "Protocol.lvclass">)
            n104 = call "Search_comm_map_and_interrogate.vi"("array of registers"=w263, "Register name"="D1", "Protocol in"=w262) -> ("output cluster"=w264:T25)  [unwired: 6 in, 2 out]
            n105 = Unbundle By Name(w264) -> ("float"=w265:sgl)
            n106 = Number To Fractional String(number=w265) -> (F-format string=w261:string)  [unwired: 3 in]
            "D1" <- w261
            n107 = Enqueue Element(queue=w270, element=ctrlCollectInfoStates."Read-D2" ("ctrlCollectInfoStates"), error in (no error)=w269) -> (error out=w268:errorcluster)  [unwired: 1 in, 2 out]
            n108 = Bundle By Name(cluster=w267, "Information.D1, 15"=w261) -> (w271:T17)
          }
          frame "Read-D2" {
            # "Next state"
            # "Read-D2 state - Reads D2"
            n109 = Unbundle By Name(w279) -> ("Comm variable definitions"=w275:T18[], "Protocol"=w274:refnum<class "Protocol.lvclass">)
            n110 = call "Search_comm_map_and_interrogate.vi"("array of registers"=w275, "Register name"="D2", "Protocol in"=w274) -> ("output cluster"=w276:T25)  [unwired: 6 in, 2 out]
            n111 = Unbundle By Name(w276) -> ("float"=w277:sgl)
            n112 = Number To Fractional String(number=w277) -> (F-format string=w273:string)  [unwired: 3 in]
            "D2" <- w273
            n113 = Enqueue Element(queue=w282, element=ctrlCollectInfoStates."Read-K1" ("ctrlCollectInfoStates"), error in (no error)=w281) -> (error out=w280:errorcluster)  [unwired: 1 in, 2 out]
            n114 = Bundle By Name(cluster=w279, "Information.D2, 16"=w273) -> (w283:T17)
          }
          frame "Read-K1" {
            # "Next state"
            # "Read-K1 state - Reads K1"
            n115 = Unbundle By Name(w291) -> ("Comm variable definitions"=w287:T18[], "Protocol"=w286:refnum<class "Protocol.lvclass">)
            n116 = call "Search_comm_map_and_interrogate.vi"("array of registers"=w287, "Register name"="K1", "Protocol in"=w286) -> ("output cluster"=w289:T25)  [unwired: 6 in, 2 out]
            n117 = Unbundle By Name(w289) -> ("float"=w290:sgl)
            n118 = Number To Fractional String(number=w290) -> (F-format string=w285:string)  [unwired: 3 in]
            "K1" <- w285
            n119 = Enqueue Element(queue=w294, element=ctrlCollectInfoStates."Read-K2" ("ctrlCollectInfoStates"), error in (no error)=w293) -> (error out=w292:errorcluster)  [unwired: 1 in, 2 out]
            n120 = Bundle By Name(cluster=w291, "Information.K1, 17"=w285) -> (w295:T17)
          }
          frame "Read-K2" {
            # "Next state"
            # "Read-K2 state - Reads K2"
            n121 = Unbundle By Name(w303) -> ("Comm variable definitions"=w298:T18[], "Protocol"=w297:refnum<class "Protocol.lvclass">)
            n122 = call "Search_comm_map_and_interrogate.vi"("array of registers"=w298, "Register name"="K2", "Protocol in"=w297) -> ("output cluster"=w300:T25)  [unwired: 6 in, 2 out]
            n123 = Unbundle By Name(w300) -> ("float"=w301:sgl)
            n124 = Number To Fractional String(number=w301) -> (F-format string=w299:string)  [unwired: 3 in]
            "K2" <- w299
            n125 = Enqueue Element(queue=w306, element=ctrlCollectInfoStates."Read-FD" ("ctrlCollectInfoStates"), error in (no error)=w305) -> (error out=w304:errorcluster)  [unwired: 1 in, 2 out]
            n126 = Bundle By Name(cluster=w303, "Information.K2, 18"=w299) -> (w307:T17)
          }
          frame "Read-FD" {
            # "Next state"
            # "Read-FD state - Reads FD"
            n127 = Unbundle By Name(w315) -> ("Comm variable definitions"=w311:T18[], "Protocol"=w310:refnum<class "Protocol.lvclass">)
            n128 = call "Search_comm_map_and_interrogate.vi"("array of registers"=w311, "Register name"="FD", "Protocol in"=w310) -> ("output cluster"=w314:T25)  [unwired: 6 in, 2 out]
            n129 = Unbundle By Name(w314) -> ("float"=w312:sgl)
            n130 = Number To Fractional String(number=w312) -> (F-format string=w309:string)  [unwired: 3 in]
            "FD" <- w309
            n131 = Enqueue Element(queue=w318, element=ctrlCollectInfoStates."Read-DenTempCoeff" ("ctrlCollectInfoStates"), error in (no error)=w317) -> (error out=w316:errorcluster)  [unwired: 1 in, 2 out]
            n132 = Bundle By Name(cluster=w315, "Information.FD, 19"=w309) -> (w319:T17)
          }
          frame "Read-DenTempCoeff" {
            # "Next state"
            # "Read-DenTempCoeff state - Reads Density Temperature Coefficient"
            n133 = Unbundle By Name(w327) -> ("Comm variable definitions"=w322:T18[], "Protocol"=w321:refnum<class "Protocol.lvclass">)
            n134 = call "Search_comm_map_and_interrogate.vi"("array of registers"=w322, "Register name"="Density Temperature Coefficient", "Protocol in"=w321) -> ("output cluster"=w324:T25)  [unwired: 6 in, 2 out]
            n135 = Unbundle By Name(w324) -> ("float"=w325:sgl)
            n136 = Number To Fractional String(number=w325) -> (F-format string=w323:string)  [unwired: 3 in]
            "Density Temp Coeff" <- w323
            n137 = Bundle By Name(cluster=w327, "Information.Density Temp Coeff, 20"=w323) -> (w331:T17)
            n138 = Enqueue Element(queue=w330, element=ctrlCollectInfoStates."Read-Srno" ("ctrlCollectInfoStates"), error in (no error)=w329) -> (error out=w328:errorcluster)  [unwired: 1 in, 2 out]
          }
          frame "Read-Srno" {
            # "Next state"
            # "Read-Srno state -  Reads Serial Number"
            n139 = Unbundle By Name(w339) -> ("Comm variable definitions"=w334:T18[], "Protocol"=w333:refnum<class "Protocol.lvclass">)
            n140 = call "Search_comm_map_and_interrogate.vi"("array of registers"=w334, "Register name"="Serial Number", "Protocol in"=w333) -> ("output cluster"=w337:T25)  [unwired: 6 in, 2 out]
            n141 = Unbundle By Name(w337) -> ("U32"=w336:u32)
            n142 = Number To Decimal String(number=w336) -> (decimal integer string=w335:string)  [unwired: 1 in]
            "Sensor Serial Number" <- w335
            n143 = Bundle By Name(cluster=w339, "Information.Transmitter Serial Number,23"=w335) -> (w343:T17)
            n144 = Enqueue Element(queue=w342, element=ctrlCollectInfoStates."Read-MassFlowUnits" ("ctrlCollectInfoStates"), error in (no error)=w341) -> (error out=w340:errorcluster)  [unwired: 1 in, 2 out]
          }
          frame "Read-MassFlowUnits" {
            # "Next state"
            # "Read-MassFlowUnits state - Reads Mass flow units"
            n145 = Unbundle By Name(w351) -> ("Comm variable definitions"=w347:T18[], "Protocol"=w346:refnum<class "Protocol.lvclass">)
            n146 = call "Search_comm_map_and_interrogate.vi"("array of registers"=w347, "Register name"="Mass flow units", "Protocol in"=w346) -> ("output cluster"=w349:T25)  [unwired: 6 in, 2 out]
            n147 = Unbundle By Name(w349) -> ("U16"=w348:u16)
            "Mass flow units" <- w348
            n148 = flat-sequence {
              tunnel: [w356] -> w345
              tunnel: w348 -> [_]
              frame #0 {
                n149 = property on="Mass flow units" class="Ring (strict)"() -> ("RingText.Text"=w356:string)  [unwired: 2 in, 2 out]
              }
            }
            n150 = Enqueue Element(queue=w354, element=ctrlCollectInfoStates."Read-DensityUnits" ("ctrlCollectInfoStates"), error in (no error)=w353) -> (error out=w352:errorcluster)  [unwired: 1 in, 2 out]
            n151 = Bundle By Name(cluster=w351, "Information.Mass Flow Units, 25"=w345) -> (w355:T17)
          }
          frame "Read-DensityUnits" {
            # "Next state"
            # "Read-DensityUnits state - Reads Density units"
            n152 = Unbundle By Name(w364) -> ("Comm variable definitions"=w360:T18[], "Protocol"=w359:refnum<class "Protocol.lvclass">)
            n153 = call "Search_comm_map_and_interrogate.vi"("array of registers"=w360, "Register name"="Density units", "Protocol in"=w359) -> ("output cluster"=w362:T25)  [unwired: 6 in, 2 out]
            n154 = Unbundle By Name(w362) -> ("U16"=w361:u16)
            "Density units" <- w361
            n155 = flat-sequence {
              tunnel: [w369] -> w358
              tunnel: w361 -> [_]
              frame #0 {
                n156 = property on="Density units" class="Ring (strict)"() -> ("RingText.Text"=w369:string)  [unwired: 2 in, 2 out]
              }
            }
            n157 = Enqueue Element(queue=w367, element=ctrlCollectInfoStates."Read-TempUnits" ("ctrlCollectInfoStates"), error in (no error)=w366) -> (error out=w365:errorcluster)  [unwired: 1 in, 2 out]
            n158 = Bundle By Name(cluster=w364, "Information.Density Units, 26"=w358) -> (w368:T17)
          }
          frame "Read-TempUnits" {
            # "Next state"
            # "Read-TempUnits state - Reads Temperature units"
            n159 = Unbundle By Name(w377) -> ("Comm variable definitions"=w373:T18[], "Protocol"=w372:refnum<class "Protocol.lvclass">)
            n160 = call "Search_comm_map_and_interrogate.vi"("array of registers"=w373, "Register name"="Temperature units", "Protocol in"=w372) -> ("output cluster"=w375:T25)  [unwired: 6 in, 2 out]
            n161 = Unbundle By Name(w375) -> ("U16"=w374:u16)
            "Temperature Units" <- w374
            n162 = flat-sequence {
              tunnel: [w382] -> w371
              tunnel: w374 -> [_]
              frame #0 {
                n163 = property on="Temperature Units" class="Ring (strict)"() -> ("RingText.Text"=w382:string)  [unwired: 2 in, 2 out]
              }
            }
            n164 = Enqueue Element(queue=w380, element=ctrlCollectInfoStates."Read-FlowCutoff" ("ctrlCollectInfoStates"), error in (no error)=w379) -> (error out=w378:errorcluster)  [unwired: 1 in, 2 out]
            n165 = Bundle By Name(cluster=w377, "Information.Temperature Units, 27"=w371) -> (w381:T17)
          }
          frame "Read-FlowCutoff" {
            # "Next state"
            # "Read-FlowCutoff state - Reads Mass flow cutoff"
            n166 = Unbundle By Name(w390) -> ("Comm variable definitions"=w386:T18[], "Protocol"=w385:refnum<class "Protocol.lvclass">)
            n167 = call "Search_comm_map_and_interrogate.vi"("array of registers"=w386, "Register name"="Mass flow cutoff", "Protocol in"=w385) -> ("output cluster"=w388:T25)  [unwired: 6 in, 2 out]
            n168 = Unbundle By Name(w388) -> ("float"=w387:sgl)
            n169 = Number To Fractional String(number=w387) -> (F-format string=w384:string)  [unwired: 3 in]
            "Mass flow cutoff" <- w384
            n170 = Enqueue Element(queue=w393, element=ctrlCollectInfoStates."Read-MassFlowDamping" ("ctrlCollectInfoStates"), error in (no error)=w392) -> (error out=w391:errorcluster)  [unwired: 1 in, 2 out]
            n171 = Bundle By Name(cluster=w390, "Information.Mass Flow Cutoff, 28"=w384) -> (w394:T17)
          }
          frame "Read-MassFlowDamping" {
            # "Next state"
            # "Read-MassFlowDamping state - Reads Flow rate internal damping"
            n172 = Unbundle By Name(w402) -> ("Comm variable definitions"=w397:T18[], "Protocol"=w396:refnum<class "Protocol.lvclass">)
            n173 = call "Search_comm_map_and_interrogate.vi"("array of registers"=w397, "Register name"="Flow rate internal damping", "Protocol in"=w396) -> ("output cluster"=w400:T25)  [unwired: 6 in, 2 out]
            n174 = Unbundle By Name(w400) -> ("float"=w399:sgl)
            n175 = Number To Fractional String(number=w399) -> (F-format string=w398:string)  [unwired: 3 in]
            "Mass flow damping" <- w398
            n176 = Bundle By Name(cluster=w402, "Information.Mass Flow Damping, 29"=w398) -> (w406:T17)
            n177 = Enqueue Element(queue=w405, element=ctrlCollectInfoStates."Read-FlowDirection" ("ctrlCollectInfoStates"), error in (no error)=w404) -> (error out=w403:errorcluster)  [unwired: 1 in, 2 out]
          }
          frame "Read-FlowDirection" {
            # "Next state"
            # "Read-FlowDirection state - Reads Flow direction"
            n178 = Unbundle By Name(w414) -> ("Comm variable definitions"=w410:T18[], "Protocol"=w409:refnum<class "Protocol.lvclass">)
            n179 = call "Search_comm_map_and_interrogate.vi"("array of registers"=w410, "Register name"="Flow direction", "Protocol in"=w409) -> ("output cluster"=w412:T25)  [unwired: 6 in, 2 out]
            n180 = Unbundle By Name(w412) -> ("U16"=w411:u16)
            "Flow direction" <- w411
            n181 = flat-sequence {
              tunnel: w411 -> [_]
              tunnel: [w419] -> w408
              frame #0 {
                n182 = property on="Flow direction" class="Ring (strict)"() -> ("RingText.Text"=w419:string)  [unwired: 2 in, 2 out]
              }
            }
            n183 = Enqueue Element(queue=w417, element=ctrlCollectInfoStates."Read-FreqFlowRate" ("ctrlCollectInfoStates"), error in (no error)=w416) -> (error out=w415:errorcluster)  [unwired: 1 in, 2 out]
            n184 = Bundle By Name(cluster=w414, "Information.Flow Direction, 30"=w408) -> (w418:T17)
          }
          frame "Read-FreqFlowRate" {
            # "Next state"
            # "Read-FreqFlowRate state - Reads Frequency/pulse output present frequency"
            n185 = Unbundle By Name(w427) -> ("Comm variable definitions"=w423:T18[], "Protocol"=w422:refnum<class "Protocol.lvclass">)
            n186 = call "Search_comm_map_and_interrogate.vi"("array of registers"=w423, "Register name"="Frequency/pulse output present frequency", "Protocol in"=w422) -> ("output cluster"=w425:T25)  [unwired: 6 in, 2 out]
            n187 = Unbundle By Name(w425) -> ("float"=w424:sgl)
            n188 = Number To Fractional String(number=w424) -> (F-format string=w421:string)  [unwired: 3 in]
            "Frequency flow rate" <- w421
            n189 = Bundle By Name(cluster=w427, "Information.Frequency Flow Rate, 31"=w421) -> (w431:T17)
            n190 = Enqueue Element(queue=w430, element=ctrlCollectInfoStates."Read-FreqSpan" ("ctrlCollectInfoStates"), error in (no error)=w429) -> (error out=w428:errorcluster)  [unwired: 1 in, 2 out]
          }
          frame "Read-FreqSpan" {
            # "Next state"
            # "Read-FreqSpan state - Reads Frequency maximum pulse width"
            n191 = Unbundle By Name(w439) -> ("Comm variable definitions"=w434:T18[], "Protocol"=w433:refnum<class "Protocol.lvclass">)
            n192 = call "Search_comm_map_and_interrogate.vi"("array of registers"=w434, "Register name"="Frequency maximum pulse width ", "Protocol in"=w433) -> ("output cluster"=w437:T25)  [unwired: 6 in, 2 out]
            n193 = Unbundle By Name(w437) -> ("float"=w436:sgl)
            n194 = Number To Fractional String(number=w436) -> (F-format string=w435:string)  [unwired: 3 in]
            "Frequency span" <- w435
            n195 = Enqueue Element(queue=w442, element=ctrlCollectInfoStates."Read-TransmitterModel" ("ctrlCollectInfoStates"), error in (no error)=w441) -> (error out=w440:errorcluster)  [unwired: 1 in, 2 out]
            n196 = Bundle By Name(cluster=w439, "Information.Frequency Span, 32"=w435) -> (w443:T17)
          }
          frame "Read-TransmitterModel" {
            # "Next state"
            # "Read-TransmitterModel state - Reads Transmitter model"
            n197 = Unbundle By Name(w451) -> ("Comm variable definitions"=w446:T18[], "Protocol"=w445:refnum<class "Protocol.lvclass">)
            n198 = call "Search_comm_map_and_interrogate.vi"("array of registers"=w446, "Register name"="Transmitter model", "Protocol in"=w445) -> ("output cluster"=w449:T25)  [unwired: 6 in, 2 out]
            n199 = Unbundle By Name(w449) -> ("U16"=w448:u16)
            n200 = Number To Decimal String(number=w448) -> (decimal integer string=w447:string)  [unwired: 1 in]
            "Transmitter Model" <- w447
            n201 = Bundle By Name(cluster=w451, "Information.Transmitter Model Number,24"=w447) -> (w455:T17)
            n202 = Enqueue Element(queue=w454, element=ctrlCollectInfoStates."Read-MeterZero" ("ctrlCollectInfoStates"), error in (no error)=w453) -> (error out=w452:errorcluster)  [unwired: 1 in, 2 out]
          }
          frame "Read-MeterZero" {
            # "Next state"
            # "Read-MeterZero state - Reads MeterZero"
            n203 = Unbundle By Name(w464) -> ("Comm variable definitions"=w458:T18[], "Protocol"=w457:refnum<class "Protocol.lvclass">)
            n204 = call "Search_comm_map_and_interrogate.vi"("array of registers"=w458, "Register name"="Meter Zero", "Protocol in"=w457) -> ("error out"=w463:errorcluster, "output cluster"=w460:T25)  [unwired: 6 in, 1 out]
            n205 = Unbundle By Name(w463) -> ("status"=→"status":bool)
            n206 = Unbundle By Name(w460) -> ("float"=w459:sgl)
            n207 = Number To Fractional String(number=w459) -> (F-format string=w456:string)  [unwired: 3 in]
            "Meter Zero" <- w456
            n208 = Enqueue Element(queue=w468, element=ctrlCollectInfoStates."ReadComplete" ("ctrlCollectInfoStates"), error in (no error)=w467) -> (error out=w466:errorcluster)  [unwired: 1 in, 2 out]
            n209 = Bundle By Name(cluster=w464, "Information.Meter Zero, 43"=w456) -> (w469:T17)
          }
          frame "ReadComplete" {
            # "Next state"
            # "ReadComplete state - Update Read Complete? status"
            n210 = Enqueue Element(queue=w475, element=ctrlCollectInfoStates."WaitforEvents" ("ctrlCollectInfoStates"), error in (no error)=w474) -> (error out=w473:errorcluster)  [unwired: 1 in, 2 out]
            n211 = Bundle By Name(cluster=w471, "Read Complete?"=TRUE) -> (w476:T17)
          }
          frame "Done&Close" {
            # "Done&Close state - Updates output"
            n212 = Unbundle By Name(w489) -> ("Read Complete?"=→"Read Completed":bool, "Information"=w490:T11)
            n213 = Equal?(x="Status *", y=enum32{"As found", "As left"}."As found") -> (x = y?=w503:bool)
            n214 = Select(t="As found" ("Technician Name*"), s=w503, f="As left") -> (s? t:f=w494:string)
            n215 = Bundle By Name(cluster=w490, "Test Comments,3"="Test Comments", "Transmitter Serial Number,23"="Transmitter Serial Number", "Sensor Model,7"="Sensor Model #", "Size,8"="Size", "Press rating, 10"="Pressure Rating", "Temp rating, 11"="Temp Rating", "Flow Accuracy, 35"="Meter flow accuracy (%) *", "Flow Repeatability, 36"="Meter flow repeatability", "Zero Stability, 37"="Meter Zero Stability (kg/min) *", "Density Accuracy, 38"="Meter Density Accuracy", "Density Repeatability, 39"="Meter Density Repeatability", "Nomincal Flow Rate, 41"="Meter Nominal Flow Rate (kg/min)*", "Customer name, 46"="Customer Name", "Customer address, 47"="Customer Address", "Sales order number, 48"="Order number", "Technician Name, 49"="Technician Name*", "ref meter, 50"="Ref meter serial number*", "Status, 45"=w494, "product code,51"="Product code*", "fluid,52"="Fluid", "fluid temp,53"="Fluid Temperature", "Customer PO, 46"="Customer PO", "Stand Uncertainty, 47"="Stand Uncertainty", "Test Gas, 48"="Test Gas", "Freq, 49"="Frequency", "Press, 50"="Pressure", "Mdot, 51"="MDOT", "Batch time, 52"="Batch Time") -> (w487:T11)
            "Information" <- w487
            n216 = Bundle By Name(cluster=w489, "Information"=w487) -> (w488:T17)
          }
        }
      }
      frame Error {
        # "Clear errors..."
        # "In case of error, clear error and continue"
        n217 = call <vilib>:"Clear Errors.vi"("error in (no error)"=w518) -> ("error out"=w517:errorcluster)  [unwired: 5 in, 1 out]
      }
    }
  }
  n218 = Release Queue(queue=w4, error in (no error)=w5) -> (error out=w7:errorcluster)  [unwired: 1 in, 2 out]
  n219 = call <vilib>:"Clear Errors.vi"("error in (no error)"=w7) -> ()  [unwired: 5 in, 2 out]
